vi "Configure Trigger (Edge).vi"(5 "Edge Slope (0: Positive)":i32(ring) items=["Positive", "Negative", "Either", "Alternate"], 6 "Filter Type (0: Off)":i32(ring) items=["Off", "High-pass Filter", "Low-pass Filter"], 7 "Input Coupling (0: AC Coupling)":i32(ring) items=["AC Coupling", "DC Coupling", "Low Frequency Reject"], 8 "error in (no error)":errorcluster, 9 "Trigger Level (0 V)":dbl, 10 "Trigger Source (0: Channel 1)":i32(ring) items=["Channel 1"=0, "Channel 2"=1, "Channel 3"=2, "Channel 4"=3, "D0"=13, "D1"=14, "D2"=15, "D3"=16, "D4"=17, "D5"=18, "D6"=19, "D7"=20, "D8"=21, "D9"=22, "D10"=23, "D11"=24, "D12"=25, "D13"=26, "D14"=27, "D15"=28, "External"=29, "Power Line"=30, "Waveform Generator"=31, "Waveform Generator1"=32, "Waveform Modulation"=33], 11 "VISA resource name":refnum<visa-resource-name>) -> (0 "error out":errorcluster, 3 "VISA resource name out":refnum<visa-resource-name>)   [LabVIEW 2015, in "Agilent 2000 3000 X-Series.lvlib"]
doc: "Configures the edge trigger mode."
uses:
  Agilent 2000 3000 X-Series.lvlib
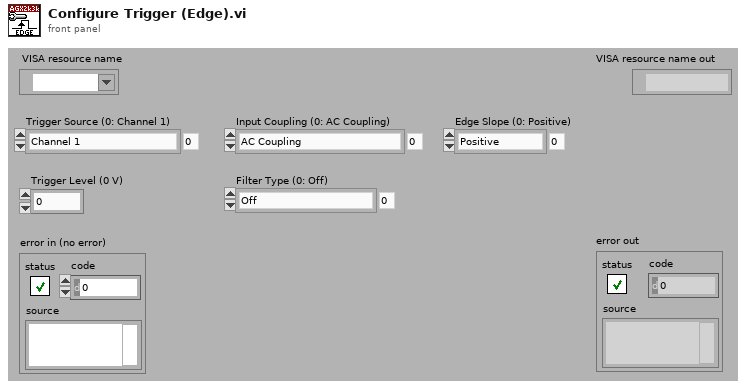
[diagram p1: front panel]
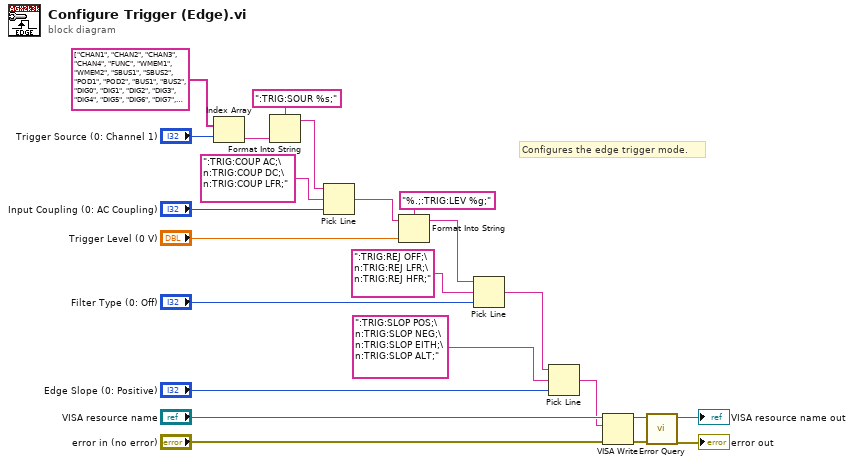
[diagram p0: block diagram]
diagram:
  # "Configures the edge trigger mode."
  n1 = Index Array(array=string[] ["CHAN1", "CHAN2", "CHAN3", "CHAN4", "FUNC", "WMEM1", "WMEM2", "SBUS1", "SBUS2", "POD1", "POD2", "BUS1", "BUS2", "DIG0", "DIG1", "DIG2", "DIG3", "DIG4", "DIG5", "DIG6", "DIG7", "DIG8", "DIG9", "DIG10", "DIG11", "DIG12", "DIG13", "DIG14", "DIG15", "EXT", "LINE", "WGEN", "WGEN1", "WMOD"], index="Trigger Source (0: Channel 1)") -> (element=w2:string)
  n2 = Format Into String(format string=":TRIG:SOUR %s;", w2) -> (resulting string=w1:string)  [unwired: 2 in, 1 out]
  n3 = Pick Line(string ("")=w1, multi-line string=":TRIG:COUP AC;\n:TRIG:COUP DC;\n:TRIG:COUP LFR;", line index="Input Coupling (0: AC Coupling)") -> (output string=w21:string)
  n4 = Format Into String(format string="%.;:TRIG:LEV %g;", initial string=w21, "Trigger Level (0 V)") -> (resulting string=w16:string)  [unwired: 1 in, 1 out]
  n5 = Pick Line(string ("")=w16, multi-line string=":TRIG:REJ OFF;\n:TRIG:REJ LFR;\n:TRIG:REJ HFR;", line index="Filter Type (0: Off)") -> (output string=w13:string)
  n6 = Pick Line(string ("")=w13, multi-line string=":TRIG:SLOP POS;\n:TRIG:SLOP NEG;\n:TRIG:SLOP EITH;\n:TRIG:SLOP ALT;", line index="Edge Slope (0: Positive)") -> (output string=w6:string)
  n7 = VISA Write(VISA resource name="VISA resource name", write buffer=w6, error in (no error)="error in (no error)") -> (VISA resource name out=w10:refnum<visa-resource-name>, error out=w9:errorcluster)  [unwired: 1 out]
  n8 = call "Error Query.vi"("error in (no error)"=w9, "VISA resource name"=w10) -> ("error out"=→"error out":errorcluster, "VISA resource name out"=→"VISA resource name out":refnum<visa-resource-name>)  [unwired: 8 out]
